vi "PID Geschwin.vi"() -> ()   [LabVIEW 2010]
panel:
  out "OUT Gesch":dbl
  in  "Rück Geschwin":dbl
  in  "Führung Geschwin":dbl
  in  "Kp Geschwin":dbl
  in  "Ki Geschwin":dbl
  in  "lower limit":dbl format="%0.2f"
  in  "upper limit":dbl format="%0.2f"
  in  "D":dbl=0.05 format="%0.2f"
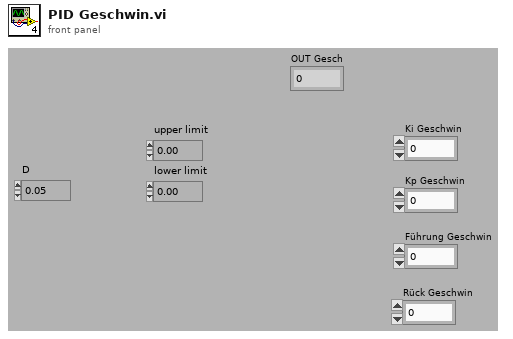
[diagram p1: front panel]
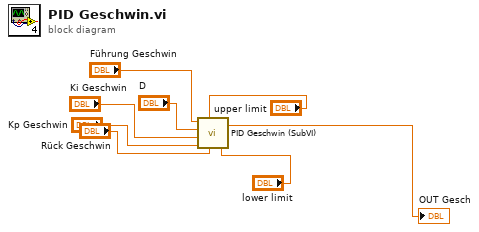
[diagram p0: block diagram]
diagram:
  n1 = call "PID Geschwin (SubVI).vi"("lower limit"="lower limit", "Rück Geschwin"="Rück Geschwin", "upper limit"="upper limit", "Kp Geschwin"="Kp Geschwin", "Ki Geschwin"="Ki Geschwin", "D"="D", "Führung Geschwin"="Führung Geschwin") -> ("OUT Gesch"=→"OUT Gesch":dbl)
